vi "subvi_analyser1boolcrossing1.vi"(8 "Action":T1=enum."Initialise", 11 "Input Bool":bool) -> (3 "Crossed?":bool)   [LabVIEW 2014]
doc: "Saves the last boolean input and compares it to the current boolean input. If the crossing Action selected occurs then returns True, else returns False."
uses:
  typedef_boolcrossing.ctl
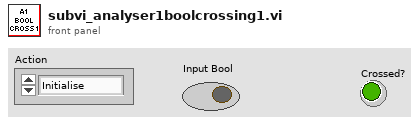
[diagram p1: front panel]
types:
  T1 = typedef "typedef_boolcrossing.ctl" = enum16{"Either", "True-False", "False-True", "Initialise"}
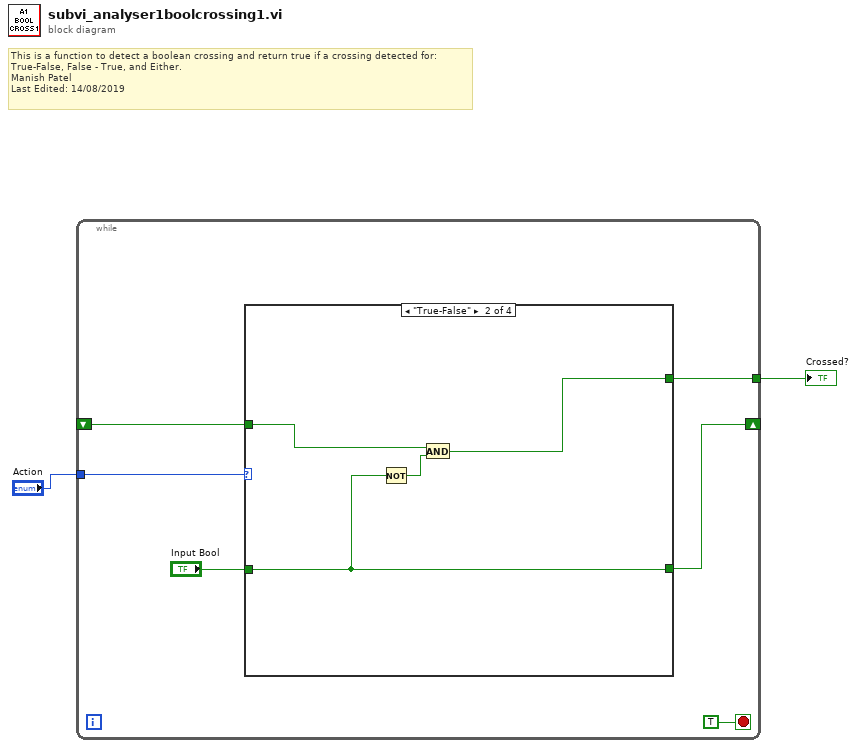
[diagram p0: block diagram]
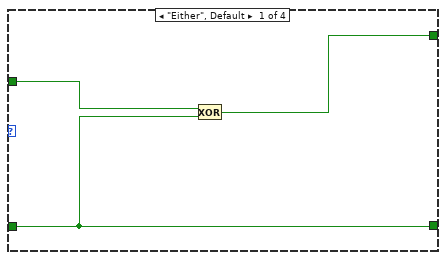
[diagram p2: hidden frame]
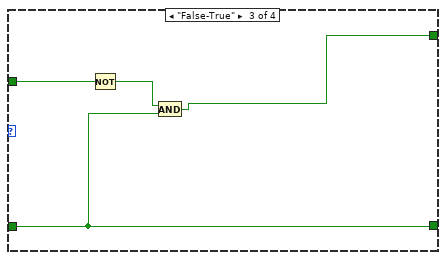
[diagram p3: hidden frame]
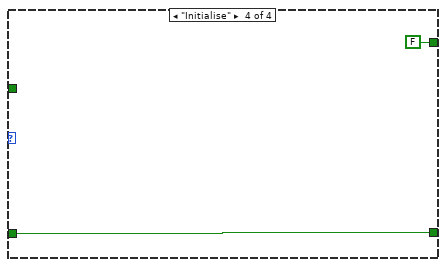
[diagram p4: hidden frame]
diagram:
  # "This is a function to detect a boolean crossing and return true if a crossing detected for:\nTrue-False, False - True, and Either.\nManish Patel\nLast Edited: 14/08/2019"
  n1 = while {
    tunnel: "Action" -> [w8]
    shift-right: [w6] -> _
    shift-left: _ -> [w5]
    tunnel: [w4] -> w1
    stop <- TRUE stop-if-true
    n2 = case shown="\"True-False\"" w8 {
      tunnel: [w11 w13 w17 w21] -> w6
      tunnel: "Input Bool" -> [w11 w13 w17 w21]
      tunnel: w5 -> [w10 w15 w19 _]
      tunnel: [w9 w12 w16 FALSE] -> w4
      frame "Either", Default {
        n3 = Exclusive Or(1:w11, 2:w10) -> (0:w9:bool)
      }
      frame "True-False" {
        n4 = Not(x=w13) -> (.not. x?=w14:bool)
        n5 = And(x=w15, y=w14) -> (x .and. y?=w12:bool)
      }
      frame "False-True" {
        n6 = Not(x=w19) -> (.not. x?=w18:bool)
        n7 = And(x=w18, y=w17) -> (x .and. y?=w16:bool)
      }
      frame "Initialise" {
      }
    }
  }
  "Crossed?" <- w1
